vi "NHMFL SCM IPS Init Sw Heater.vi"(0 "VISA session":refnum<visa-resource-name>) -> (1 "dup VISA session":refnum<visa-resource-name>, 2 "Persistent Field":dbl=1.0 format="%.2f")   [LabVIEW 2019]
panel:
  out "Persistent Field":dbl format="%.6g"
  out "String Read":string
  in  "OK Button":bool
  # "The switch heater is off!\nThe power supply indicates that the \nmagnet is persistent at the field indicated below.\nIf that is correct please hit OK.\nIf you are not sure please get help from mK personnel"
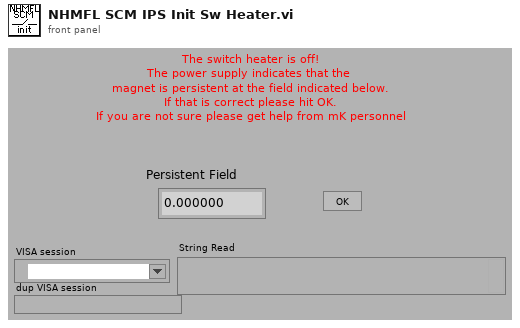
[diagram p1: front panel]
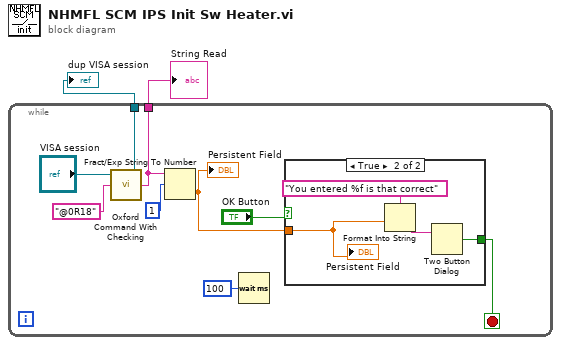
[diagram p0: block diagram]
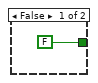
[diagram p2: hidden frame]
diagram:
  n1 = while {
    tunnel: [w6] -> w2
    tunnel: [w3] -> w1
    stop <- w10 stop-if-true
    n2 = call "Oxford Command With Checking.vi"("Command"="@0R18", "VISA session"="VISA session") -> ("String Read"=w6:string, "dup VISA session"=w3:refnum<visa-resource-name>)  [unwired: 1 in, 1 out]
    n3 = Fract/Exp String To Number(string=w6, offset=1) -> (number=w4:dbl)  [unwired: 2 in, 1 out]
    "Persistent Field" <- w4
    n4 = Wait (ms)(milliseconds to wait=u32 100) -> ()  [unwired: 1 out]
    n5 = case shown="True" "OK Button" {
      tunnel: [FALSE w14] -> w10
      tunnel: w4 -> [_ w13]
      frame False {
      }
      frame True {
        n6 = Format Into String(format string="You entered %f is that correct", w13) -> (resulting string=w16:string)  [unwired: 2 in, 1 out]
        n7 = Two Button Dialog(message=w16) -> (T button?=w14:bool)  [unwired: 2 in]
        "Persistent Field" <- w13
      }
    }
  }
  "String Read" <- w2
  "dup VISA session" <- w1
